vi "Periodic Tasks Cheeto.vi"(8 "error in":errorcluster) -> ()   [LabVIEW 2016]
doc: "This VI runs in parallel to other tasks. It can contain as many user-defined periodic loops as you need. These can carry out PID or other sorts of timed response."
uses:
  Fault_Cluster.ctl
  Faults.ctl
  <vilib>/Platform/TimedLoop/XDataNode/timing_clust.ctl
  <vilib>/Platform/TimedLoop/XDataNode/nitl_modes.ctl
  <vilib>/Platform/TimedLoop/XDataNode/wakeup.ctl
  <vilib>/Rock Robotics/SystemInterfaces/DIO/FPGA_DIOChannel.ctl
  <userlib>/836-libraries/Drive/Drive_Code/Drive_Code_Support/Drive_Code_PID_Bundle.ctl
  <vilib>/Rock Robotics/WPI/ThirdParty/CanMotor/TalonSRX/WPI_CANTalonSRX_APIFeedbackSelect.ctl
  <vilib>/Rock Robotics/WPI/ThirdParty/CanMotor/TalonSRX/WPI_CANTalonSRX_APIControlMode.ctl
  <vilib>/Rock Robotics/WPI/Utilities/WPI_GetSetVariantRefNum.vi
  <vilib>/platform/TimedLoop/XDataNode/XDataNode.xnode
  <vilib>/Platform/TimedLoop/XDataNode/XDNodeRunTimeDep.lvlib
panel:
  out "TurretLate?":bool
  out "Motor Output":dbl=-0.0
  out "Finished Late? [i-1]":bool
  in  "Period":i64=50
  in  "Log Top":bool
  out "Bot Current 2":dbl(graph)=3.75
  in  "Bottom Shooter Wheel Tab":T1(tab)=enum."Turret"
  in  "Tab Control 3":enum32{"TBH", "PID(F)"}(tab)
  in  "Bot Average":u8=10 min=1 max=128
  in  "Bot Min Rate":dbl=20.0
  in  "Bot tbh Gain":dbl
  in  "Enc Counts 3":dbl=4096.0
  in  "FF":bool=TRUE
  out "State":bool=TRUE
  out "Iter":i32=18978
  in  "delay":i32=30
  in  "FF Gain":dbl=0.000182 format="%#_13g"
  in  "Ramp Rate 3":dbl
  in  "I Zone 3":dbl
  in  "F 3":dbl=0.0288
  in  "D 3":dbl=5.0
  in  "I 3":dbl=0.001
  in  "P 3":dbl=0.19
  in  "Rev FB Sensor":bool=TRUE
  in  "Enc Counts":dbl=4096.0
  out "Bot Response":cluster{"Bot Cntrl":dbl, dbl}(graph)={"Bot Cntrl"=0.0, 2145.6268149735524}
  in  "Bot Cntrl":dbl(knob)=2145.6268149735524 scale=0.0..5700.0
  in  "BotInvert":bool=TRUE
  in  "Bot Period":i64=15
  in  "Disable Bottom":bool
  out "Bot Late?":bool
  in  "Bot Tol":dbl=25.0 format="%#_13g"
  out "RPM High .":bool
  out "RPM Low .":bool=TRUE
  out "1 RPM .":bool
  out "5 RPM .":bool
  out "2 RPM .":bool
  out "8 RPM .":bool
  out "7 RPM .":bool
  out "6 RPM .":bool
  out "4 RPM .":bool
  out "3 RPM .":bool
  out "RPM Steady? 2":bool
  in  "Open?":bool=TRUE
  out "Bot Cntrl .":dbl=2145.6268149735524
  in  "Log Bot Current?":bool
  out "Max Bot":dbl=0.29296875
  in  "reset bot":bool
  out "Min Bot":dbl=-0.146484375
  out "Stopped":bool=TRUE
  out "Bot Dist":dbl=67108856.0
  in  "Open Loop Cntrl":dbl(knob)=0.0014346101200435335 scale=-1.0..1.0
  out "Tgrd 2":bool
  out "cnt 2":i16=90
  in  "Arm2":bool=TRUE
  in  "Trig2":dbl=40.0
  in  "Len2":i16=90
  in  "Reset2":bool
  out "State2":i32
  out "File Delete Checking":string
  in  "LogTR":bool
  in  "LogTL":bool
  in  "LogBL":bool
  in  "LogBR":bool
  in  "TR":T2 {"Severity" max=10}
  in  "BR":T2 {"Severity" max=10}
  in  "BL":T2 {"Severity" max=10}
  in  "TL":T2 {"Severity" max=10}
  out "Turret":cluster{"Double":dbl, "desired Angle":dbl}(graph)={"Double"=0.29942691101875774, "desired Angle"=0.0}
  in  "Invert Turret":bool
  in  "Turret Max Speed":dbl(knob)=0.618529087034838 scale=0.0..1.0
  in  "SoftStop":bool=TRUE
  in  "correlation":bool
  out "At Lo":bool
  out "At Hi":bool=TRUE
  in  "Lo Limit":dbl=-70.0
  in  "Hi Limit":dbl=40.0
  in  "Speed near Limit":dbl=0.2
  in  "Near Limit":dbl=40.0
  out "Motor Out":dbl
  out "Angle":dbl
  in  "PID gains":T4={"proportional gain (Kc)"=0.02, "integral time (Ti, min)"=0.0, "derivative time (Td, min)"=0.001} {"derivative time (Td, min)" format="%.3f"; "integral time (Ti, min)" format="%.8f"; "proportional gain (Kc)" format="%.8f"}
  in  "output range":cluster{"output high":dbl, "output low":dbl}={"output high"=1.0, "output low"=-1.0}
  in  "shooter range":dbl=100.0 format="%#_13g"
  in  "Softstop":dbl
  in  "desired Angle":dbl(slide) scale=-100.0..90.0
  in  "Out Bound":dbl=100.0
  in  "Track Target":bool
  in  "Soft Stop Period":dbl(knob) scale=0.0..1.0
  in  "Manual":bool=TRUE
  in  "Soft Stops":T5={"Motor Power"=0.0, "Time to Stop"=0.0, "Hi Limit"=95.0, "Lo Limit"=-90.0, "Speed Near Limit"=0.15, "Near Limit"=35.0}
  in  "Tolerance":dbl
  out "TtR":dbl
  out "Tgrd 3":bool
  out "cnt 3":i16=90
  in  "Arm 2":bool=TRUE
  in  "Trig 2":dbl=20.0
  in  "Len 2":i16=90
  in  "Reset1 2":bool
  out "State1 2":i32
  in  "Invert Primer":bool
  in  "Primer Max Speed":dbl(knob)=1.0 scale=0.0..1.0
  in  "Invert Agitator":bool
  in  "Agitator Max Speed":dbl(knob)=1.0 scale=0.0..1.0
  in  "Invert Intake":bool
  in  "Intake Speed":dbl(knob)=1.0 scale=0.0..1.0
  out "Roll":dbl(graph)=-2.653997926222683
  out "Pitch":dbl(graph)=0.9060832058624935
  out "Yaw":dbl(graph)=64.04836303793759
  out "Yaw Alt":dbl(graph)=1.0254433926321722
  out "Pitch Alt":dbl(graph)=3.179870559290271
  out "Roll Alt":dbl(graph)=14.748416919967577
  in  "Top Shooter Wheel Tab":T6(tab)=enum."Control"
  in  "Tab Control 2":enum32{"TBH", "PID(F)"}(tab)=enum."PID(F)"
  in  "switch pnt":dbl=2800.0
  in  "Top Gain (lower)":dbl=6e-06
  in  "Top Gain (upper)":dbl=2e-05
  in  "Top Min Rate":dbl=20.0
  in  "Top Average":u8=30 min=1 max=128
  in  "P 2":dbl=0.075 format="%#_8g"
  in  "I 2":dbl=0.001
  in  "D 2":dbl=5.0
  in  "F 2":dbl=0.0132
  in  "I Zone 2":dbl
  in  "Ramp Rate 2":dbl
  in  "Enc Counts 2":dbl=4096.0
  in  "Rev FB Sensor 2":bool=TRUE
  out "Top Cntrl .":dbl=-3139.2166644166086
  in  "Top Cntrl":dbl(knob)=-3139.2166644166086 scale=-7000.0..7000.0
  out "Top Response":cluster{"Top Cntrl":dbl, dbl}(graph)={"Top Cntrl"=0.0, -3139.2166644166086}
  in  "TopInvert":bool
  in  "Top Period":i64=17
  in  "Disable Top":bool
  out "RPM Steady? Top":bool
  out "3 RPM":bool
  out "4 RPM":bool
  out "6 RPM":bool
  out "7 RPM":bool
  out "8 RPM":bool
  out "2 RPM":bool
  out "5 RPM":bool
  out "1 RPM":bool
  out "RPM Low":bool
  out "RPM High":bool=TRUE
  in  "Top Tol":dbl=25.0 format="%#_13g"
  out "Top Late?":bool
  in  "reset top":bool
  out "Max top":dbl=0.43945312499999994
  out "Min Top":dbl=-0.732421875
  out "Stopped 2":bool=TRUE
  out "Top Dist":dbl=-67108864.0
  out "Tgrd":bool
  out "cnt":i16=90
  in  "Arm":bool=TRUE
  in  "Trig":dbl=20.0
  in  "Len":i16=90
  in  "Reset1":bool
  out "State1":i32
  in  "Top Open":bool=TRUE
  in  "Output":dbl(knob) scale=0.0..10.0
  out "appended path":path
  out "TDMS Name":string="Shooter Log"
  in  "Log to USB?":bool
  in  "TDMS Name 2":string="Shooter Log"
  out "File Creation Loop Iteration":i32
  in  "Burst 2":i32=75
  out "Save Drive 2":bool=TRUE
  out "Save Drive":bool
  in  "Burst":i32=75
  in  "loop period (ms) 2":u32=200
  out "Bot Current":dbl(graph)=3.0
  out "Top Current":dbl(graph)
  in  "Bot Channel":i32=14
  in  "Top Channel":i32=13
  in  "Bot Channel 2":i32=2
  # "Start"
  # "Top Wheel"
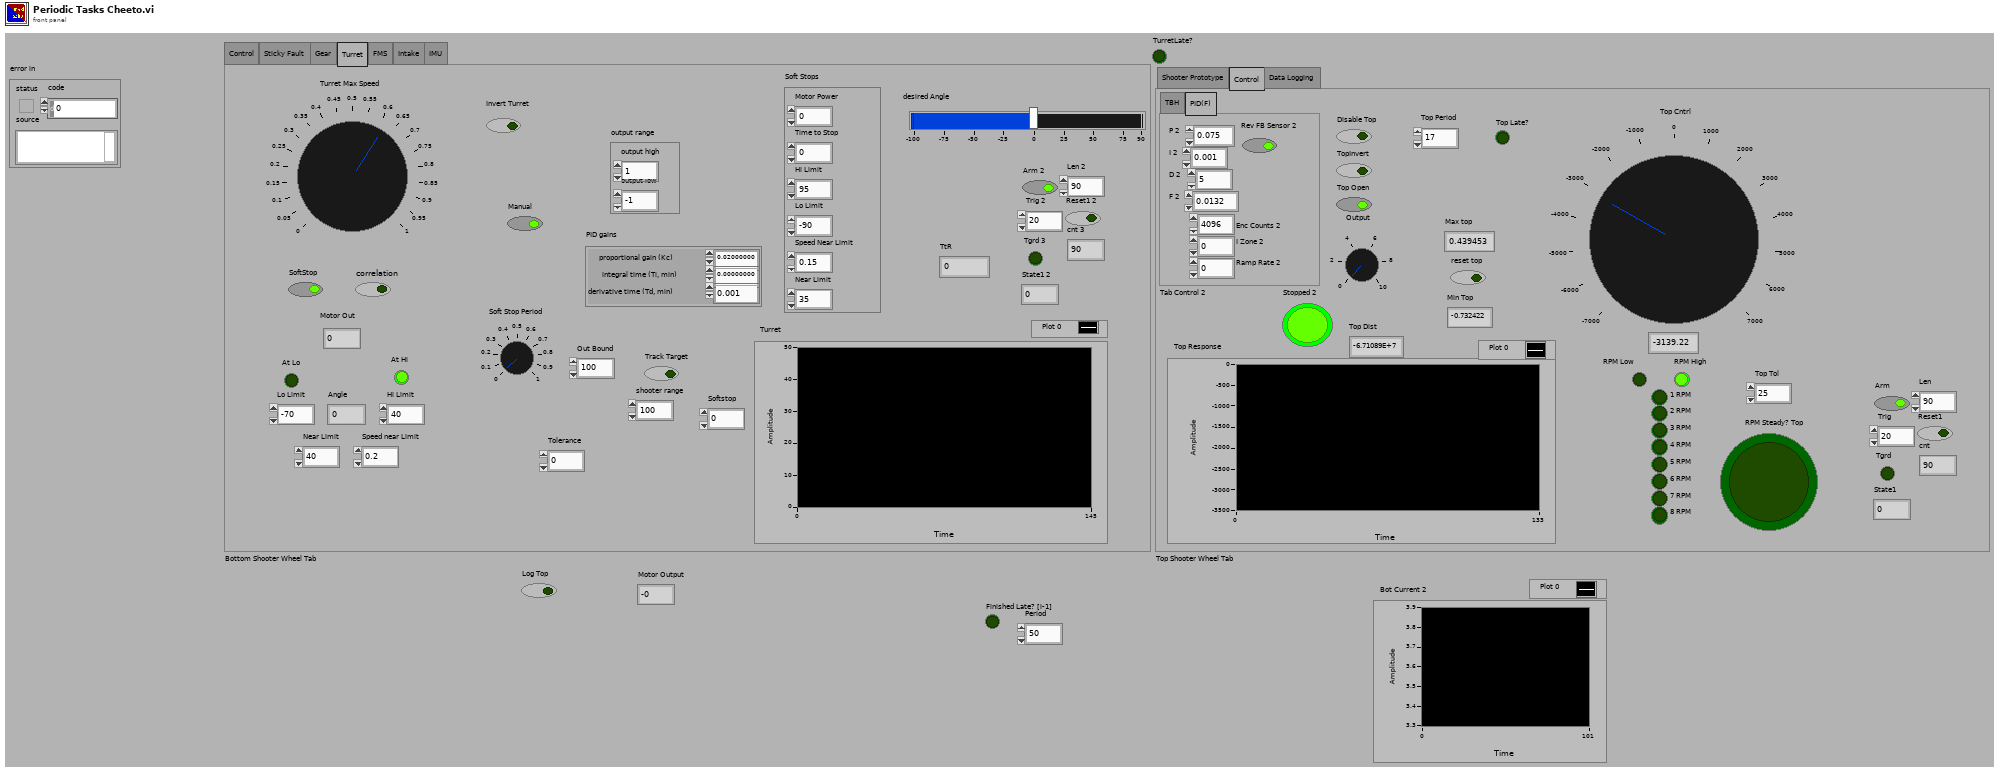
[diagram p1: front panel]
types:
  T1 = enum32{"Control", "Sticky Fault", "Gear", "Turret", "FMS", "Intake", "IMU"}
  T2 = typedef "Fault_Cluster.ctl" = cluster{"Error Code":T3, "Severity":u32, "Message":string, "Origin":string}
  T3 = typedef "Faults.ctl" = enum16{"Boiler Target Lost", "Gerar Target Lost", "Body IMU Fault", "Turret IMU Fault"}
  T4 = cluster{"proportional gain (Kc)":dbl, "integral time (Ti, min)":dbl, "derivative time (Td, min)":dbl}
  T5 = cluster{"Motor Power":dbl, "Time to Stop":dbl, "Hi Limit":dbl, "Lo Limit":dbl, "Speed Near Limit":dbl, "Near Limit":dbl}
  T6 = enum32{"Shooter Prototype", "Control", "Data Logging"}
  T7 = typedef "FPGA_DIOChannel.ctl" = enum8{"DIO 0", "DIO 1", "DIO 2", "DIO 3", "DIO 4", "DIO 5", "DIO 6", "DIO 7", "DIO 8", "DIO 9", "DIO MXP 0", "DIO MXP 1", "DIO MXP 2", "DIO MXP 3", "DIO MXP 4", "DIO MXP 5", "DIO MXP 6", "DIO MXP 7", "DIO MXP 8", "DIO MXP 9", "DIO MXP 10", "DIO MXP 11", "DIO MXP 12", "DIO MXP 13", "DIO MXP 14", "DIO MXP 15", "SPI Port CS1", "SPI Port CS2", "SPI Port CS3", "SPI Port MISO", "SPI Port MOSI", "Invalid"}
  T8 = typedef "XDNodeRunTimeDep.lvlib/timing_clust.ctl" = cluster{"Expected End [f-1]":u64, "Actual End [f-1]":u64, "Finished Late? [f-1]":bool, "Expected End [i-1]":u64, "Actual End [i-1]":u64, "Finished Late? [i-1]":bool, "Expected Start [i]":u64, "Actual Start [i]":u64, "Expected Start [f]":u64, "Actual Start [f]":u64, "Source Name":string, "Structure Name":string, "Period":i64, "Deadline":i64, "Offset":i64, "Start":i64, "Priority":i32, "Timeout":i32, "Mode":T9, "Wakeup Reason":T10, "Error":errorcluster, "Source Type":string, "Secondary Source Type":string, "Global End Time":u64, "Global Start Time":u64, "Frame Duration":u64, "Iteration Duration":u64, "Assigned CPU":i32, "I/O Scan Engine Mode":u32}
  T9 = typedef "XDNodeRunTimeDep.lvlib/nitl_modes.ctl" = enum32{"No Change", "Process missed periods, maintain original phase", "Discard missed periods, maintain original phase", "Process missed periods, ignore original phase", "Discard missed periods, ignore original phase"}
  T10 = typedef "XDNodeRunTimeDep.lvlib/wakeup.ctl" = enum32{"Normal", "Aborted", "Asynchronous wakeup", "Timing source error", "Timed loop error", "Timeout"}
  T11 = typedef "Fault_Fifos.ctl" = cluster{"Error Code":refnum<k33>, "Severity":refnum<k33>, "Burst":refnum<k4>, "BurstSize":u32, "Timing Notifier":refnum<notifier>, "Timing Trigger":u16}
  T12 = enum16{"open", "open or create", "create or replace", "create", "open (read-only)"}
  T13 = typedef "WPI_MotorControlDeviceRef.ctl" = cluster{"DeviceStatus":errorcluster, "Type":T14, "PWM":cluster{"PWM Channel":T15, "DeadBand":T16}, "CAN":cluster{"Device Number":u8, "SetOutput VI Ref":variant, "GetOutput VI Ref":variant, "Enable VI Ref":variant, "Disable VI Ref":variant, "Data":variant}, "Invert":bool}
  T14 = typedef "WPI_MotorControlType.ctl" = enum16{"PWM", "CAN"}
  T15 = typedef "FPGA_DIOPWMChannel.ctl" = enum8{"PWM 0", "PWM 1", "PWM 2", "PWM 3", "PWM 4", "PWM 5", "PWM 6", "PWM 7", "PWM 8", "PWM 9", "PWM MXP 0", "PWM MXP 1", "PWM MXP 2", "PWM MXP 3", "PWM MXP 4", "PWM MXP 5", "PWM MXP 6", "PWM MXP 7", "PWM MXP 8", "PWM MXP 9", "Invalid"}
  T16 = typedef "WPI_PWMDeadband.ctl" = cluster{"Name":string, "maxPositivePwm":i32, "minPositivePwm":i32, "centerPwm":i32, "maxNegativePwm":i32, "minNegativePwm":i32, "angularRange":u16}
  T17 = typedef "WPI_EncoderDevRef.ctl" = cluster{"DevStatus":errorcluster, "EncoderIndex":T18, "CounterIndex":T19, "DistancePerCount":dbl, "Decoding Type":T20}
  T18 = typedef "FPGA_EncoderIdx.ctl" = enum8{"Enc 0", "Enc 1", "Enc 2", "Enc 3", "Enc 4", "Enc 5", "Enc 6", "Enc 7", "Invalid"}
  T19 = typedef "FPGA_CounterCtrSystemIndex.ctl" = enum8{"Ctr 0", "Ctr 1", "Ctr 2", "Ctr 3", "Ctr 4", "Ctr 5", "Ctr 6", "Ctr 7", "Invalid"}
  T20 = typedef "WPI_EncoderType.ctl" = enum16{"1x", "2x", "4x"}
  T21 = typedef "WPI_CANTalonSRX_APIFeedbackSelect.ctl" = enum16{"Digital Quadrature Encoder", "Analog Potentiometer", "Analog Encoder", "Count on Quad-A (Rising-Edge)", "Count on Quad-A (Falling-Edge)", "CTR Magnetic Enc (Absolute)", "CTR Magnetic Enc (Relative)", "Pulse Width"}
  T22 = typedef "WPI_CANTalonSRX_APIControlMode.ctl" = enum8{"Percent VBus", "Speed", "Position", "Slave", "Unchanged / Invalid", "Voltage Compensation", "Current", "Motion Profile", "Motion Magic"}
  T23 = typedef "WPI_CANTalonSRX_GlobalStatus.ctl" = cluster{"Applied Throttle":dbl, "Module Enabled":bool, "CAN Error":errorcluster, "Closed Loop Error":dbl, "Forward Limit Switch Closed":bool, "Reverse Limit Switch Closed":bool, "Sensor Position":dbl, "Sensor Velocity":dbl, "Current":dbl, "Sticky Fault - Over Temp":bool, "Sticky Fault - Under Voltage":bool, "Sticky Fault - Forward Limit":bool, "Sticky Fault - Reverse Limit":bool, "Sticky Fault - Forward Soft Limit":bool, "Sticky Fault - Reverse Soft Limit":bool, "Brake is Enabled":bool, "Encoder Position":dbl, "Encoder Velocity":dbl, "Encoder Index Count":dbl, "Encoder A Pin State":bool, "Encoder B Pin State":bool, "Encoder Index Pin State":bool, "Analog In":dbl, "Analog In Velocity":dbl, "Temperature (C)":dbl, "Battery Voltage":dbl, "Control 5 Is Supported":bool, "Current Profile Slot Select":dbl, "Pos Div 8":bool, "Vel Div 4":bool, "Pulse Width Position":i32, "Pulse Width Velocity":i32, "Pulse Width Rise To Rise (us)":i32, "Pulse Width Rise To Fall (us)":i32, "Mot Prof Active Is Under Run":bool, "Mot Prof Active Has Under Run":bool, "Mot Prof Active Is Last":bool, "Mot Prof Active Velocity Only":bool, "Mot Prof Active Is Valid":bool, "Mot Prof Buffer Is Full":bool, "Mot Prof Active Profile Slot Select":i32, "Mot Prof NextID":i32, "Mot Prof Count":i32, "Mot Prof Active Velocity":dbl, "Mot Prof Active Position":dbl, "Mot Prof Output Enable":i32}
  T24 = typedef "WPI_JoystickDevRef.ctl" = cluster{"Device":T25}
  T25 = typedef "WPI_JoystickDeviceEnum.ctl" = enum16{"USB 0", "USB 1", "USB 2", "USB 3", "USB 4", "USB 5"}
  T26 = typedef "WPI_DigitalInputDevRef.ctl" = cluster{"DevStatus":errorcluster, "DIO Channel":T7}
  T27 = typedef "WPI_I2CDevRef.ctl" = cluster{"DevStatus":errorcluster, "Device Address":u8, "Handle":i32, "I2C Bus":T28}
  T28 = typedef "i2c_bus.ctl" = enum16{"I2C On-Board", "I2C MXP", "Invalid"}
  T29 = cluster{"Yaw":dbl, "Roll":dbl, "Pitch":dbl, "Yaw Wind":dbl, "Roll Wind":dbl, "Pitch Wind":dbl}
  T30 = typedef "WPI_RobotDriveDevRef.ctl" = cluster{"DevStatus":errorcluster, "Motors[]":T13[], "Square Inputs":bool, "Max Output":dbl}
  T31 = typedef "Drive_Code_Bundle.ctl" = cluster{"Sensor Data":T32, "Drive Command rt fifo":refnum<k33>, "Logging Data":refnum<k33>, "PID Update":refnum<notifier>}
  T32 = typedef "Sensor_Cluster.ctl" = cluster{"Gyro Data":cluster{"Gyro RT FIFO":refnum<k33>, "Gyro Current":dbl, "Gyro Hold":dbl}, "Encoder Data":cluster{"Encoder RT FIFO":refnum<k33>, "Encoder Current":dbl, "Encoder Hold":dbl}, "Camera Data":cluster{"Camera RT FIFO":refnum<k33>, "Camera Current":T33}}
  T33 = typedef "Camera_Cluster.ctl" = cluster{" Angle":dbl, "Valid":bool}
  T34 = typedef "Drive_Code_PID_Bundle.ctl" = cluster{"Yaw, Driving Straight":cluster{"proportional gain (Kc)":dbl, "integral time (Ti, min)":dbl, "derivative time (Td, min)":dbl}, "Yaw, Holding Still":cluster{"proportional gain (Kc)":dbl, "integral time (Ti, min)":dbl, "derivative time (Td, min)":dbl}, "Distance, Driving Straight":cluster{"proportional gain (Kc)":dbl, "integral time (Ti, min)":dbl, "derivative time (Td, min)":dbl}, "Distance, Holding Still":cluster{"proportional gain (Kc)":dbl, "integral time (Ti, min)":dbl, "derivative time (Td, min)":dbl}}
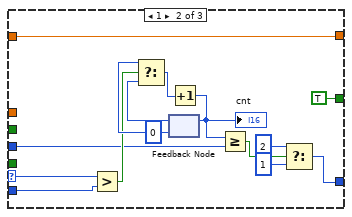
[diagram p3: hidden frame]
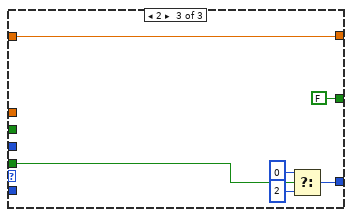
[diagram p4: hidden frame]
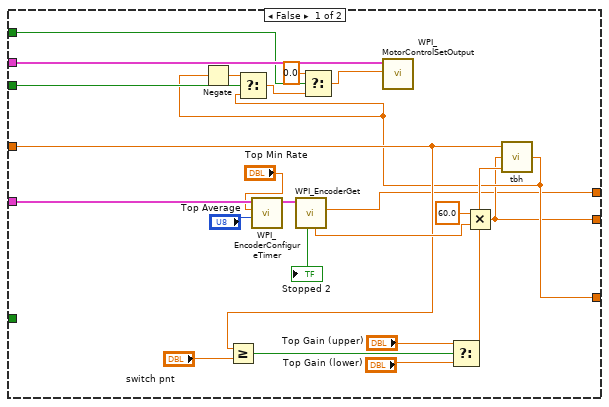
[diagram p6: hidden frame]
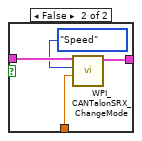
[diagram p7: hidden frame]
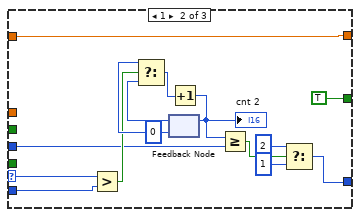
[diagram p9: hidden frame]
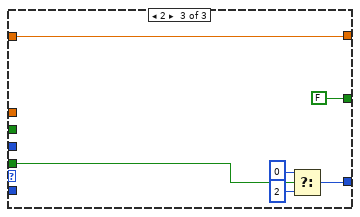
[diagram p10: hidden frame]
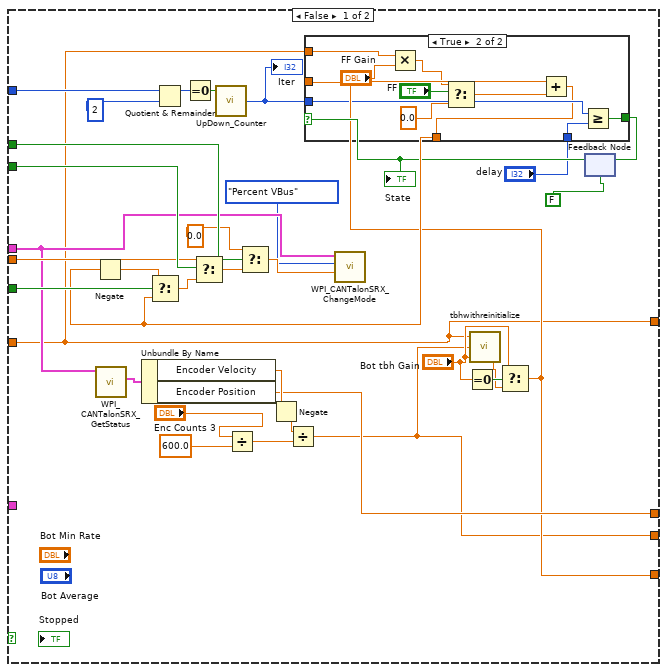
[diagram p11: hidden frame]
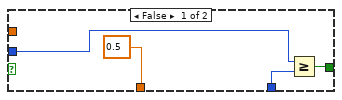
[diagram p12: hidden frame]
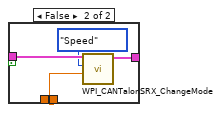
[diagram p14: hidden frame]
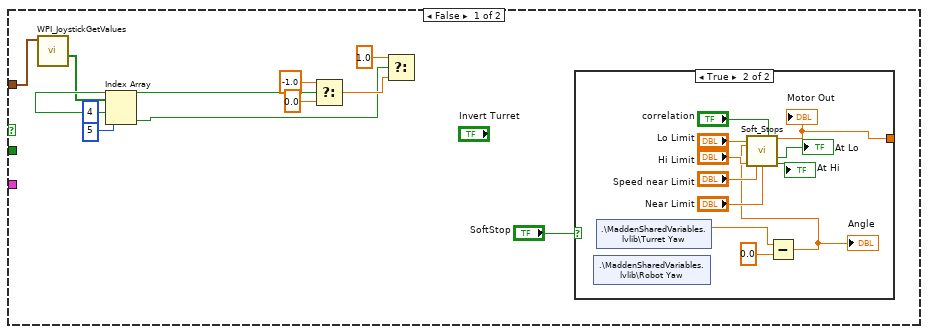
[diagram p16: hidden frame]
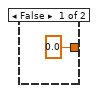
[diagram p17: hidden frame]
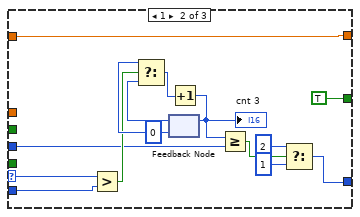
[diagram p19: hidden frame]
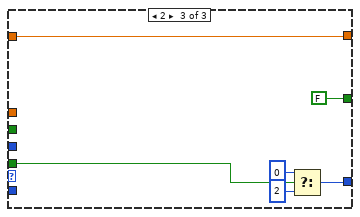
[diagram p20: hidden frame]
diagram:
  # "Drive FIFO Setup"
  # "rising edges\none channel only\nspeed control"
  n1 = disable-structure shown="Disabled" {
    disable-tunnel: [w55 _] -> w48
    frame Disabled {
      n2 = while {
        tunnel: [w68] -> w55
        tunnel: "Log to USB?" -> [w57]
        tunnel: "TDMS Name 2" -> [w56]
        i -> [w72]
        stop <- w69 continue-if-true
        # "Can tweak this such that it doesn't start until Time > 1970"
        n3 = Current VI's Path() -> (path=w67:path)
        n4 = Strip Path(path=w67) -> (stripped path=w61:path)  [unwired: 1 out]
        n5 = String To Path(string="~/") -> (path=w65:path)
        n6 = Select(t=w65, s=w57, f=w61) -> (s? t:f=w66:path)
        n7 = Get Date/Time In Seconds() -> (seconds since 1Jan1904=w74:timestamp)
        n8 = case shown="False" w57 {
          selector: w57 -> [w80 _]
          tunnel: w66 -> [w79 w85]
          tunnel: [w79 w82] -> w63
          tunnel: [w80 w81] -> w60
          frame False {
          }
          frame True {
            n9 = Build Path(base path=w85, name or relative path="LogFiles") -> (appended path=w84:path)
            n10 = call <vilib>:"Check if File or Folder Exists.vi"("path"=w84) -> ("file or folder exists?"=w88:bool, "dup path"=w87:path)  [unwired: 8 in, 1 out]
            n11 = case shown="False" w88 {
              tunnel: [w90 w91] -> w83
              tunnel: w87 -> [w89 w91]
              frame False {
                n12 = Create Folder(path (use dialog)=w89) -> (created path=w90:path)  [unwired: 2 in, 2 out]
              }
              frame True {
              }
            }
            n13 = call <vilib>:"Check if File or Folder Exists.vi"("path"=w83) -> ("file or folder exists?"=w81:bool, "dup path"=w82:path)  [unwired: 8 in, 1 out]
          }
        }
        n14 = Format Date/Time String(time format string (%c)="%m-%#d-%Y %H%M", seconds (now)=w74, UTC format=FALSE) -> (date/time string=w77:string)
        n15 = Number To Hexadecimal String(1:i16 4 ("width (-)"), 2:w72) -> (0:w70:string)
        n16 = Concatenate Strings(w56, w77, w70, ".tdms" ("string")) -> (w78:string)
        n17 = case shown="True" w60 {
          tunnel: w61 -> [w96 w101]
          tunnel: [w92 w101] -> w59
          frame False {
            n18 = Build Path(base path=w96, name or relative path="LogFiles") -> (appended path=w93:path)
            n19 = call <vilib>:"Check if File or Folder Exists.vi"("path"=w93) -> ("file or folder exists?"=w94:bool, "dup path"=w95:path)  [unwired: 8 in, 1 out]
            n20 = case shown="False" w94 {
              tunnel: [w99 w100] -> w92
              tunnel: w95 -> [w98 w100]
              frame False {
                n21 = Create Folder(path (use dialog)=w98) -> (created path=w99:path)  [unwired: 2 in, 2 out]
              }
              frame True {
              }
            }
          }
          frame True {
          }
        }
        n22 = Select(t=w63, s=w60, f=w59) -> (s? t:f=w62:path)
        n23 = Build Path(base path=w62, name or relative path=w78) -> (appended path=w68:path)
        n24 = call <vilib>:"Check if File or Folder Exists.vi"("path"=w68) -> ("file or folder exists?"=w69:bool)  [unwired: 8 in, 2 out]
        n25 = Wait (ms)(milliseconds to wait=u32 1 ("millisecond multiple")) -> ()  [unwired: 1 out]
        "File Creation Loop Iteration" <- w72
      }
      n26 = disable-structure shown="Disabled" {
        frame Disabled {
          w109 = i64 50 ("Period")
          # "needs testing"
          # "Periodic Data Log Setup"
          n27 = Obtain Notifier(name (unnamed)="Timing", notification data type=u16 0) -> (notifier out=w105:refnum<notifier>)  [unwired: 2 in, 2 out]
          n28 = call "OpenFaultLogger.vi"("Timing Trigger"=u16 1, "Timing Notifier"=w105, "BurstSize"=u32 4, "BufferSize"=u32 100) -> ("FaultDevRef"=w102:T11)  [unwired: 7 in]
          n29 = node-c288(w109) -> (w118:T8)  [unwired: 3 in]
          n30 = node-c288(w109) -> (w112:T8)  [unwired: 3 in]
          n31 = timed-loop {
            timing: w118 -> [_]
            timing-out: [_] -> w117
            tunnel: w102 -> [w151]
            stop <- FALSE stop-if-true
            n32 = node-c288() -> ()  [unwired: 1 in, 1 out]
            n33 = call "WriteFault.vi"("Fault"="TL", "FaultDevRef"=w151) -> ()  [unwired: 1 in]
            n34 = while {
              stop <- "LogTL" stop-if-true
            }
            n35 = node-c288() -> ()  [unwired: 1 in, 1 out]
          }
          n36 = timed-loop {
            timing: w112 -> [_]
            timing-out: [_] -> w111
            tunnel: w102 -> [w121]
            stop <- FALSE stop-if-true
            n37 = node-c288() -> ()  [unwired: 1 in, 1 out]
            n38 = while {
              stop <- "LogBL" stop-if-true
            }
            n39 = call "WriteFault.vi"("Fault"="BL", "FaultDevRef"=w121) -> ()  [unwired: 1 in]
            n40 = node-c288() -> ()  [unwired: 1 in, 1 out]
          }
          n41 = node-c288(w117) -> ()  [unwired: 1 out]
          n42 = node-c288(w111) -> ()  [unwired: 1 out]
          n43 = call "FaultLogger.vi"("Period"=i64 20, "FaultDevRef"=w102) -> ()  [unwired: 10 in]
          n44 = node-c288(w109) -> (w114:T8)  [unwired: 3 in]
          n45 = node-c288(w109) -> (w116:T8)  [unwired: 3 in]
          n46 = timed-loop {
            timing: w114 -> [_]
            timing-out: [_] -> w113
            tunnel: w102 -> [w131]
            stop <- FALSE stop-if-true
            n47 = node-c288() -> ()  [unwired: 1 in, 1 out]
            n48 = while {
              stop <- "LogBR" stop-if-true
            }
            n49 = call "WriteFault.vi"("Fault"="BR", "FaultDevRef"=w131) -> ()  [unwired: 1 in]
            n50 = node-c288() -> ()  [unwired: 1 in, 1 out]
          }
          n51 = timed-loop {
            timing: w116 -> [_]
            timing-out: [_] -> w115
            tunnel: w102 -> [w141]
            stop <- FALSE stop-if-true
            n52 = node-c288() -> ()  [unwired: 1 in, 1 out]
            n53 = call "WriteFault.vi"("Fault"="TR", "FaultDevRef"=w141) -> ()  [unwired: 1 in]
            n54 = while {
              stop <- "LogTR" stop-if-true
            }
            n55 = node-c288() -> ()  [unwired: 1 in, 1 out]
          }
          n56 = node-c288(w113) -> ()  [unwired: 1 out]
          n57 = node-c288(w115) -> ()  [unwired: 1 out]
        }
        frame Enabled {
        }
      }
    }
    frame Enabled {
    }
  }
  "appended path" <- w48
  n58 = disable-structure shown="Disabled" {
    frame Disabled {
      n59 = node-c288(i64 100 ("Period")) -> (w161:T8)  [unwired: 3 in]
      n60 = timed-loop {
        timing: w161 -> [_]
        timing-out: [_] -> w160
        stop <- FALSE stop-if-true
        w162 = 1.0 ("Secondary True Time")
        # "needs verified"
        # "0: delete file\n1: ask if sure\n2: don't do anything"
        # "Sticky Fault File Deletion"
        n61 = node-c288() -> ()  [unwired: 1 in, 1 out]
        n62 = call <vilib>:"WPI_UtilitiesFRC ReadUserButton.vi"() -> ("User Button"=w176:bool)  [unwired: 10 in, 1 out]
        n63 = call <userlib>:"BoolConfirmCheck.vi"("False Time"=3.0, "Secondary True Time"=w162, "Inital True Time"=5.0, "Signal"=w176) -> ("First Time Met"=w172:bool, "Out Signal"=w173:bool)
        n64 = call <userlib>:"Pulse_Stretch_&_Delay.vi"("In"=w172, "Width (sec)"=w162) -> ("Out"=w164:bool)  [unwired: 3 in]
        n65 = call <userlib>:"Pulse_Stretch_&_Delay.vi"("In"=w173, "Width (sec)"=w162) -> ("Out"=w163:bool)  [unwired: 3 in]
        n66 = Select(t=1, s=w164, f=2) -> (s? t:f=w168:i32)
        n67 = Select(t=0, s=w163, f=w168) -> (s? t:f=w166:i32)
        n68 = case shown="1" w166 {
          tunnel: ["File Deleted" "Ask if Sure" "Nothing Done To File"] -> w165
          frame 0 {
          }
          frame 1 {
          }
          frame 2, Default {
          }
        }
        "File Delete Checking" <- w165
        n69 = node-c288() -> ()  [unwired: 1 in, 1 out]
      }
      n70 = node-c288(w160) -> ()  [unwired: 1 out]
    }
    frame Enabled {
    }
  }
  n71 = disable-structure shown="Disabled" {
    disable-tunnel: w48 -> [w187 _]
    frame Disabled {
      w198 = 9 ("dimension size")
      # "Size of Drive Log"
      # "13"
      n72 = TDMS Open(6:TRUE ("disable buffering? (T)"), 7:enum16{"1.0", "2.0"}."2.0" ("file format version (2.0)"), 10:T12."open or create" ("operation (0:open)"), 11:w187) -> (3:w192:refnum<k34>)  [unwired: 3 in, 1 out]
      n73 = Initialize Array(0.0, w198) -> (w188:dbl[])
      n74 = To Unsigned Long Integer(number=w198) -> (unsigned 32bit integer=w199:u32)
      n75 = RT FIFO Create(0:"Drive FIFO" ("name (unnamed)"), 1:w188, 4:u32 100 ("size (10)"), 6:w199) -> (8:w190:refnum<k33>)  [unwired: 4 in, 2 out]
      n76 = while "Drive Logging Loop" {
        tunnel: w190 -> [w239]
        tunnel: w188 -> [w238]
        tunnel: w192 -> [w237]
        stop <- FALSE stop-if-true
        n77 = local read "Save Drive 2"() -> (w235:bool)
        n78 = local read "Burst 2"() -> (w233:i32)
        n79 = disable-structure shown="Disabled" {
          disable-tunnel: w239 -> [w244 _]
          disable-tunnel: w238 -> [w243 _]
          disable-tunnel: w237 -> [w242 _]
          disable-tunnel: w235 -> [w241 _]
          disable-tunnel: w233 -> [w240 _]
          frame Disabled {
            n80 = call "Drive Data Logger.vi"("Save"=w241, "Array"=w243, "Burst"=w240, "rt fifo"=w244, "TDMS Refnum"=w242) -> ()  [unwired: 7 in]
          }
          frame Enabled {
          }
        }
        n81 = Wait (ms)(milliseconds to wait="loop period (ms) 2") -> ()  [unwired: 1 out]
      }
      n82 = Get Date/Time In Seconds() -> (seconds since 1Jan1904=w191:timestamp)
      n83 = To Double Precision Float(number=w191) -> (double precision float=w189:dbl)
      n84 = while {
        tunnel: w190 -> [w212]
        tunnel: w188 -> [w211]
        tunnel: w189 -> [w210]
        stop <- FALSE stop-if-true
        n85 = shared-variable ".\\Untitled Library 1.lvlib\\Control Signal1"() -> (w209:dbl)  [unwired: 1 in, 1 out]
        n86 = shared-variable ".\\Untitled Library 1.lvlib\\Current1"() -> (w208:dbl)  [unwired: 1 in, 1 out]
        n87 = shared-variable ".\\Untitled Library 1.lvlib\\Rpm1"() -> (w207:dbl)  [unwired: 1 in, 1 out]
        n88 = shared-variable ".\\Untitled Library 1.lvlib\\Control Signal2"() -> (w206:dbl)  [unwired: 1 in, 1 out]
        n89 = shared-variable ".\\Untitled Library 1.lvlib\\Current2"() -> (w205:dbl)  [unwired: 1 in, 1 out]
        n90 = shared-variable ".\\Untitled Library 1.lvlib\\Rpm2"() -> (w204:dbl)  [unwired: 1 in, 1 out]
        n91 = shared-variable ".\\Untitled Library 1.lvlib\\Current3"() -> (w200:dbl)  [unwired: 1 in, 1 out]
        n92 = case shown="True" TRUE {
          tunnel: w211 -> [_ w228]
          tunnel: w210 -> [_ w227]
          tunnel: w212 -> [_ w226]
          tunnel: w209 -> [_ w221]
          tunnel: w208 -> [_ w220]
          tunnel: w207 -> [_ w219]
          tunnel: w206 -> [_ w218]
          tunnel: w205 -> [_ w217]
          tunnel: w204 -> [_ w216]
          tunnel: w200 -> [_ w214]
          frame False {
          }
          frame True {
            n93 = Get Date/Time In Seconds() -> (seconds since 1Jan1904=w231:timestamp)
            n94 = To Double Precision Float(number=w231) -> (double precision float=w232:dbl)
            n95 = Subtract(x=w232, y=w227) -> (x-y=w222:dbl)
            n96 = feedback #1(u32 0 ("# elements")) -> (w215:u32)
            n97 = Replace Array Subset(array=w228, new element #1=w222, new element #2=w221, new element #3=w220, new element #4=w219, new element #5=w218, new element #6=w217, new element #7=w216, new element #8=w214, new element #9=w215) -> (w229:dbl[])  [unwired: 9 in]
            n98 = RT FIFO Write(0:w226, 1:w229) -> (7:w225:u32)  [unwired: 3 in, 3 out]
            n99 = feedback-in #1(w225) -> ()
            n100 = Greater?(x=w225, y="Burst 2") -> (0:→"Save Drive 2":bool)
          }
        }
        n101 = Wait (ms)(milliseconds to wait=u32 20) -> ()  [unwired: 1 out]
        n102 = Wait (ms)(milliseconds to wait=u32 40) -> ()  [unwired: 1 out]
      }
    }
    frame Enabled {
    }
  }
  n103 = call <vilib>:"WPI_MotorControlRefNum Registry Get.vi"("refnum name"="TopMotor") -> ("MotorControlDevRef"=w1:T13)  [unwired: 9 in, 1 out]
  n104 = call <vilib>:"WPI_EncoderRefNum Registry Get.vi"("refnum name"="TopWheelSpeed") -> ("EncoderDevRef"=w2:T17)  [unwired: 9 in, 1 out]
  n105 = node-c288() -> (w6:T8)  [unwired: 5 in]
  n106 = timed-loop {
    timing: w6 -> [_]
    timing-out: [_] -> w5
    tunnel: w2 -> [w300]
    tunnel: w1 -> [w302]
    stop <- FALSE stop-if-true
    w261 = 0.0
    n107 = node-c288() -> (→"Top Late?":bool)  [unwired: 1 in, 1 out]
    n108 = case shown="True" "Log Top" {
      frame False {
      }
      frame True {
        n109 = call <vilib>:"WPI_Power Get PDP Currents.vi"("PDP Channel"="Top Channel") -> ("current (A)"=w354:dbl)  [unwired: 12 in, 2 out]
        "Top Current" <- w354
        n110 = shared-variable ".\\Untitled Library 1.lvlib\\Current2"(w354) -> ()  [unwired: 1 in, 1 out]
      }
    }
    n111 = case shown="True" TRUE {
      tunnel: w302 -> [w378 w389]
      tunnel: w300 -> [w376 _]
      tunnel: "TopInvert" -> [w373 _]
      tunnel: "Disable Top" -> [w367 _]
      tunnel: "Top Cntrl" -> [w360 w385]
      tunnel: [w359 w387] -> w271
      tunnel: [w357 w379] -> w246
      tunnel: [w356 w388] -> w259
      tunnel: "Top Open" -> [_ w380]
      frame False {
        n112 = Greater Or Equal?(x=w360, y="switch pnt") -> (x >= y?=w361:bool)
        n113 = call <vilib>:"WPI_EncoderConfigureTimer.vi"("Number Samples to Average"="Top Average", "Minimum Rate"="Top Min Rate", "EncoderDevRef"=w376) -> ("EncoderDevRef"=w377:T17)  [unwired: 7 in, 1 out]
        n114 = call <vilib>:"WPI_EncoderGet.vi"("EncoderDevRef"=w377) -> ("Distance"=w356:dbl, "Rate"=w371:dbl, "Stopped"=→"Stopped 2":bool)  [unwired: 5 in, 3 out]
        n115 = Select(t="Top Gain (upper)", s=w361, f="Top Gain (lower)") -> (s? t:f=w363:dbl)
        n116 = Multiply(x=60.0 ("y"), y=w371) -> (x*y=w357:dbl)
        n117 = call "tbh.vi"("Gain"=w363, "Act"=w357, "Cmd"=w360) -> ("Out"=w359:dbl)
        n118 = Negate(x=w359) -> (-x=w372:dbl)
        n119 = Select(t=w372, s=w373, f=w359) -> (s? t:f=w369:dbl)
        n120 = Select(t=0.0, s=w367, f=w369) -> (s? t:f=w368:dbl)
        n121 = call <vilib>:"WPI_MotorControlSetOutput.vi"("Output"=w368, "MotorControlDevRef"=w378) -> ()  [unwired: 7 in, 3 out]
      }
      frame True {
        n122 = call <vilib>:"WPI_CANTalonSRX_SetReference.vi"("Reverse Feedback Sensor"="Rev FB Sensor 2", "Feedback Reference"=WPI_CANTalonSRX_APIFeedbackSelect."Digital Quadrature Encoder", "CAN Talon SRX Ref"=w389) -> ("CAN Talon SRX Ref"=w401:T13)  [unwired: 7 in, 1 out]
        n123 = Divide(x="Enc Counts 2", y=600.0) -> (x/y=w390:dbl)
        n124 = Multiply(x=w390, y=w385) -> (x*y=w383:dbl)
        n125 = call <vilib>:"WPI_CANTalonSRX_SetPID.vi"("CAN Talon SRX Ref"=w401, "Parameter Slot"=u8 0, "P"="P 2", "I"="I 2", "D"="D 2", "F"="F 2", "I Zone"="I Zone 2", "Ramp Rate"="Ramp Rate 2") -> ("CAN Talon SRX Ref"=w403:T13)  [unwired: 6 in, 1 out]
        n126 = Negate(x=w383) -> (-x=w381:dbl)
        n127 = case shown="True" w380 {
          tunnel: w403 -> [w407 w411]
          tunnel: [w406 w410] -> w402
          tunnel: w381 -> [_ w408]
          frame True {
            n128 = call <vilib>:"WPI_CANTalonSRX_ChangeMode.vi"("Output"="Output", "Control Mode"=WPI_CANTalonSRX_APIControlMode."Percent VBus", "CAN Talon SRX Ref"=w407) -> ("CAN Talon SRX Ref"=w406:T13)  [unwired: 7 in, 1 out]
          }
          frame False {
            n129 = call <vilib>:"WPI_CANTalonSRX_ChangeMode.vi"("Output"=w408, "Control Mode"=WPI_CANTalonSRX_APIControlMode."Speed", "CAN Talon SRX Ref"=w411) -> ("CAN Talon SRX Ref"=w410:T13)  [unwired: 7 in, 1 out]
          }
        }
        n130 = call <vilib>:"WPI_CANTalonSRX_GetStatus.vi"("CAN Talon SRX Ref"=w402) -> ("Talon SRX Status"=w400:T23)  [unwired: 8 in, 2 out]
        n131 = Unbundle By Name(w400) -> ("Encoder Velocity"=w386:dbl, "Applied Throttle"=w387:dbl, "Encoder Position"=w388:dbl)
        n132 = Divide(x=w386, y=w390) -> (x/y=w379:dbl)
      }
    }
    "Top Dist" <- w259
    n133 = feedback #2(w261) -> (w269:dbl)
    n134 = Select(t=-inf, s="reset top", f=w269) -> (s? t:f=w268:dbl)
    n135 = Max & Min(x=w246, y=w268) -> (max(x,y)=w270:dbl)  [unwired: 1 out]
    "Max top" <- w270
    n136 = feedback-in #2(w270) -> ()
    n137 = shared-variable ".\\Untitled Library 1.lvlib\\Rpm2"(w246) -> ()  [unwired: 1 in, 1 out]
    n138 = Bundle("Top Cntrl"="Top Cntrl", w246) -> ()  [unwired: 1 in, 1 out]
    n139 = shared-variable ".\\Untitled Library 1.lvlib\\Control Signal2"(w271) -> ()  [unwired: 1 in, 1 out]
    n140 = feedback #3(w261) -> (w264:dbl)
    n141 = Select(t=inf, s="reset top", f=w264) -> (s? t:f=w266:dbl)
    n142 = Max & Min(x=w246, y=w266) -> (min(x,y)=w265:dbl)  [unwired: 1 out]
    "Min Top" <- w265
    n143 = feedback-in #3(w265) -> ()
    n144 = Add(x="Top Cntrl", y="Top Tol") -> (x+y=w276:dbl)
    n145 = Subtract(x="Top Cntrl", y="Top Tol") -> (x-y=w275:dbl)
    n146 = Subtract(x="Top Cntrl", y=w246) -> (x-y=w296:dbl)
    n147 = Less Than 0?(x=w296) -> (x < 0?=→"RPM High":bool)
    n148 = Greater Than 0?(x=w296) -> (x > 0?=→"RPM Low":bool)
    n149 = Absolute Value(x=w296) -> (abs(x)=w293:dbl)
    n150 = In Range and Coerce(upper limit=w276, x=w246, lower limit=w275) -> (In Range?=→"RPM Steady? Top":bool)  [unwired: 1 out]
    n151 = Less Or Equal?(x=w293, y=1.0) -> (x <= y?=→"1 RPM":bool)
    n152 = Less Or Equal?(x=w293, y=2.0) -> (x <= y?=→"2 RPM":bool)
    n153 = Less Or Equal?(x=w293, y=3.0) -> (x <= y?=→"3 RPM":bool)
    n154 = Less Or Equal?(x=w293, y=4.0) -> (x <= y?=→"4 RPM":bool)
    n155 = Less Or Equal?(x=w293, y=5.0) -> (x <= y?=→"5 RPM":bool)
    n156 = Less Or Equal?(x=w293, y=6.0) -> (x <= y?=→"6 RPM":bool)
    n157 = Less Or Equal?(x=w293, y=7.0) -> (x <= y?=→"7 RPM":bool)
    n158 = Less Or Equal?(x=w293, y=8.0) -> (x <= y?=→"8 RPM":bool)
    n159 = feedback #4(0) -> (w252:i32)
    "State1" <- w252
    n160 = feedback #5(w252) -> (w251:i32)
    n161 = feedback-in #5(w252) -> ()
    n162 = case shown="0, Default" w252 {
      selector: w252 -> [w309 w344 _]
      tunnel: w246 -> [w315 w335 w353]
      tunnel: [w331 w339 w352] -> w249
      tunnel: "Arm" -> [w330 _ _]
      tunnel: "Trig" -> [w311 _ _]
      tunnel: w251 -> [w310 w343 _]
      tunnel: "Len" -> [_ w341 _]
      tunnel: [w315 w335 w353] -> w256
      tunnel: "Reset1" -> [w307 _ w349]
      tunnel: [TRUE TRUE FALSE] -> w255
      frame 0, Default {
        w329 = 0
        n163 = Less?(x=w309, y=w310) -> (x < y?=w308:bool)
        n164 = Or(x=w307, y=w308) -> (x .or. y?=w306:bool)
        n165 = feedback #6(-inf) -> (w321:dbl)
        n166 = Select(t=w315, s=w306, f=w321) -> (s? t:f=w320:dbl)
        n167 = Max & Min(x=w315, y=w320) -> (max(x,y)=w327:dbl)  [unwired: 1 out]
        n168 = feedback-in #6(w327) -> ()
        n169 = feedback #7(inf) -> (w319:dbl)
        n170 = Select(t=w315, s=w306, f=w319) -> (s? t:f=w318:dbl)
        n171 = Max & Min(x=w315, y=w318) -> (min(x,y)=w326:dbl)  [unwired: 1 out]
        n172 = Add(x=w326, y=w327) -> (x+y=w325:dbl)
        n173 = Divide(x=w325, y=2.0) -> (x/y=w314:dbl)
        n174 = feedback-in #7(w326) -> ()
        n175 = Add(x=w311, y=w314) -> (x+y=w317:dbl)
        n176 = Subtract(x=w314, y=w311) -> (x-y=w316:dbl)
        n177 = In Range and Coerce(upper limit=w317, x=w315, lower limit=w316) -> (In Range?=w313:bool)  [unwired: 1 out]
        n178 = Not(x=w313) -> (.not. x?=w312:bool)
        "Tgrd" <- w312
        n179 = Select(t=1, s=w312, f=w329) -> (s? t:f=w332:i32)
        n180 = Select(t=w332, s=w330, f=w329) -> (s? t:f=w331:i32)
      }
      frame 1 {
        w346 = i16 0
        n181 = Greater?(x=w344, y=w343) -> (0:w342:bool)
        n182 = feedback #8(w346) -> (w347:i16)
        n183 = Select(t=w346, s=w342, f=w347) -> (s? t:f=w345:i16)
        n184 = Increment(x=w345) -> (x+1=w340:i16)
        "cnt" <- w340
        n185 = feedback-in #8(w340) -> ()
        n186 = Greater Or Equal?(x=w340, y=w341) -> (x >= y?=w336:bool)
        n187 = Select(t=2, s=w336, f=1) -> (s? t:f=w339:i32)
      }
      frame 2 {
        n188 = Select(t=0, s=w349, f=2) -> (s? t:f=w352:i32)
      }
    }
    n189 = feedback-in #4(w249) -> ()
    n190 = case shown="True" w255 {
      tunnel: w256 -> [_ w305]
      tunnel: "Top Cntrl" -> [_ w303]
      frame False {
      }
      frame True {
        n191 = Bundle(w305, "Top Cntrl"=w303) -> (→"Top Response":cluster{dbl, "Top Cntrl":dbl})  [unwired: 1 in]
      }
    }
    n192 = node-c288("Top Period") -> ()  [unwired: 1 in, 1 out]
    "Top Cntrl ." <- "Top Cntrl"
  }
  n193 = call <vilib>:"WPI_EncoderRefNum Registry Get.vi"("refnum name"="BottomWheelSpeed") -> ("EncoderDevRef"=w52:T17)  [unwired: 9 in, 1 out]
  n194 = call <vilib>:"WPI_MotorControlRefNum Registry Get.vi"("refnum name"="BottomMotor") -> ("MotorControlDevRef"=w51:T13)  [unwired: 9 in, 1 out]
  n195 = node-c288(w5) -> ()  [unwired: 1 out]
  n196 = node-c288() -> (w8:T8)  [unwired: 4 in]
  n197 = timed-loop {
    timing: w8 -> [_]
    timing-out: [_] -> w7
    tunnel: w52 -> [w474]
    tunnel: w51 -> [w476]
    i -> [w442]
    stop <- FALSE stop-if-true
    w433 = -inf
    w432 = inf
    n198 = node-c288() -> (→"Bot Late?":bool)  [unwired: 1 in, 1 out]
    n199 = case shown="True" TRUE {
      tunnel: w476 -> [w537 w597]
      tunnel: w474 -> [_ _]
      tunnel: "BotInvert" -> [w561 _]
      tunnel: "Bot Cntrl" -> [w530 w581]
      tunnel: "Disable Bottom" -> [w557 _]
      tunnel: "Open?" -> [w556 w580]
      tunnel: "Open Loop Cntrl" -> [w555 w579]
      tunnel: [w532 w586] -> w443
      tunnel: w442 -> [w546 _]
      tunnel: [w529 w578] -> w418
      tunnel: [w530 w581] -> w417
      tunnel: [w538 w582] -> w430
      frame False {
        n200 = call <vilib>:"WPI_CANTalonSRX_GetStatus.vi"("CAN Talon SRX Ref"=w537) -> ("Talon SRX Status"=w540:T23)  [unwired: 8 in, 2 out]
        n201 = Unbundle By Name(w540) -> ("Encoder Velocity"=w539:dbl, "Encoder Position"=w538:dbl)
        n202 = Quotient & Remainder(x=w546, y=2) -> (x-y*floor(x/y)=w548:i32)  [unwired: 1 out]
        n203 = Equal To 0?(x=w548) -> (x = 0?=w547:bool)
        n204 = call <userlib>:"UpDown_Counter.vi"("up"=w547) -> ("count"=w545:i32)  [unwired: 4 in]
        "Iter" <- w545
        n205 = Divide(x="Enc Counts 3", y=600.0) -> (x/y=w541:dbl)
        n206 = Negate(x=w539) -> (-x=w534:dbl)
        n207 = Divide(x=w534, y=w541) -> (x/y=w529:dbl)
        n208 = Equal To 0?(x="Bot tbh Gain") -> (x = 0?=w533:bool)
        n209 = call "tbhwithreinitialize.vi"("Gain"="Bot tbh Gain", "Act"=w529, "Cmd"=w530) -> ("Out"=w528:dbl)
        n210 = Select(t="Bot tbh Gain", s=w533, f=w528) -> (s? t:f=w532:dbl)
        n211 = feedback #9(FALSE) -> (w551:bool)
        "State" <- w551
        n212 = case shown="True" w551 {
          tunnel: [0.5 w572] -> w553
          tunnel: w532 -> [_ w573]
          tunnel: [w564 w576] -> w552
          tunnel: w545 -> [w563 w574]
          tunnel: "delay" -> [w562 w575]
          tunnel: w530 -> [_ w568]
          frame False {
            n213 = Greater Or Equal?(x=w563, y=w562) -> (x >= y?=w564:bool)
          }
          frame True {
            n214 = Multiply(x=w568, y="FF Gain") -> (x*y=w567:dbl)
            n215 = Select(t=w567, s="FF", f=0.0) -> (s? t:f=w571:dbl)
            n216 = Add(x=w573, y=w571) -> (x+y=w572:dbl)
            n217 = Greater Or Equal?(x=w574, y=w575) -> (x >= y?=w576:bool)
          }
        }
        n218 = Negate(x=w553) -> (-x=w560:dbl)
        n219 = Select(t=w560, s=w561, f=w553) -> (s? t:f=w559:dbl)
        n220 = Select(t=w555, s=w556, f=w559) -> (s? t:f=w558:dbl)
        n221 = Select(t=0.0, s=w557, f=w558) -> (s? t:f=w536:dbl)
        n222 = call <vilib>:"WPI_CANTalonSRX_ChangeMode.vi"("Output"=w536, "Control Mode"=WPI_CANTalonSRX_APIControlMode."Percent VBus", "CAN Talon SRX Ref"=w537) -> ()  [unwired: 7 in, 2 out]
        n223 = feedback-in #9(w552) -> ()
      }
      frame True {
        n224 = call <vilib>:"WPI_CANTalonSRX_SetReference.vi"("Reverse Feedback Sensor"="Rev FB Sensor", "Feedback Reference"=WPI_CANTalonSRX_APIFeedbackSelect."Digital Quadrature Encoder", "CAN Talon SRX Ref"=w597) -> ("CAN Talon SRX Ref"=w601:T13)  [unwired: 7 in, 1 out]
        n225 = Divide(x="Enc Counts", y=600.0) -> (x/y=w589:dbl)
        n226 = Multiply(x=w589, y=w581) -> (x*y=w585:dbl)
        n227 = call <vilib>:"WPI_CANTalonSRX_SetPID.vi"("CAN Talon SRX Ref"=w601, "P"="P 3", "I"="I 3", "D"="D 3", "F"="F 3", "I Zone"="I Zone 3", "Ramp Rate"="Ramp Rate 3") -> ("CAN Talon SRX Ref"=w603:T13)  [unwired: 7 in, 1 out]
        n228 = Negate(x=w585) -> (-x=w584:dbl)
        n229 = case shown="True" w580 {
          tunnel: w603 -> [w607 w611]
          tunnel: [w606 w610] -> w602
          tunnel: w584 -> [_ w608]
          tunnel: w579 -> [w604 _]
          frame True {
            n230 = call <vilib>:"WPI_CANTalonSRX_ChangeMode.vi"("Output"=w604, "Control Mode"=WPI_CANTalonSRX_APIControlMode."Percent VBus", "CAN Talon SRX Ref"=w607) -> ("CAN Talon SRX Ref"=w606:T13)  [unwired: 7 in, 1 out]
          }
          frame False {
            n231 = call <vilib>:"WPI_CANTalonSRX_ChangeMode.vi"("Output"=w608, "Control Mode"=WPI_CANTalonSRX_APIControlMode."Speed", "CAN Talon SRX Ref"=w611) -> ("CAN Talon SRX Ref"=w610:T13)  [unwired: 7 in, 1 out]
          }
        }
        n232 = disable-structure shown="Disabled" {
          frame Disabled {
            n233 = call "RPM2FF.vi"() -> ()  [unwired: 11 in, 1 out]
          }
          frame Enabled {
          }
        }
        n234 = call <vilib>:"WPI_CANTalonSRX_GetStatus.vi"("CAN Talon SRX Ref"=w602) -> ("Talon SRX Status"=w600:T23)  [unwired: 8 in, 2 out]
        n235 = Unbundle By Name(w600) -> ("Encoder Velocity"=w588:dbl, "Applied Throttle"=w586:dbl, "Encoder Position"=w582:dbl)
        n236 = Negate(x=w588) -> (-x=w583:dbl)
        n237 = Divide(x=w583, y=w589) -> (x/y=w587:dbl)
        n238 = Negate(x=w587) -> (-x=w578:dbl)
      }
    }
    "Bot Cntrl ." <- w417
    "Bot Dist" <- w430
    n239 = case shown="True" "Log Bot Current?" {
      frame False {
      }
      frame True {
        n240 = call <vilib>:"WPI_Power Get PDP Currents.vi"("PDP Channel"="Bot Channel") -> ("current (A)"=w614:dbl)  [unwired: 12 in, 2 out]
        "Bot Current" <- w614
        n241 = shared-variable ".\\Untitled Library 1.lvlib\\Current1"(w614) -> ()  [unwired: 1 in, 1 out]
        n242 = call <vilib>:"WPI_Power Get PDP Currents.vi"("PDP Channel"="Bot Channel 2") -> ("current (A)"=w613:dbl)  [unwired: 12 in, 2 out]
        "Bot Current 2" <- w613
        n243 = shared-variable ".\\Untitled Library 1.lvlib\\Current3"(w613) -> ()  [unwired: 1 in, 1 out]
      }
    }
    n244 = Bundle("Bot Cntrl"=w417, w418) -> ()  [unwired: 1 in, 1 out]
    n245 = Add(x=w417, y="Bot Tol") -> (x+y=w467:dbl)
    n246 = Subtract(x=w417, y="Bot Tol") -> (x-y=w468:dbl)
    n247 = feedback #10(w433) -> (w439:dbl)
    n248 = Select(t=w433, s="reset bot", f=w439) -> (s? t:f=w438:dbl)
    n249 = shared-variable ".\\Untitled Library 1.lvlib\\Rpm1"(w418) -> ()  [unwired: 1 in, 1 out]
    n250 = shared-variable ".\\Untitled Library 1.lvlib\\Control Signal1"(w443) -> ()  [unwired: 1 in, 1 out]
    n251 = Subtract(x=w417, y=w418) -> (x-y=w447:dbl)
    n252 = Max & Min(x=w418, y=w438) -> (max(x,y)=w440:dbl)  [unwired: 1 out]
    "Max Bot" <- w440
    n253 = feedback-in #10(w440) -> ()
    n254 = Less Than 0?(x=w447) -> (x < 0?=→"RPM High .":bool)
    n255 = Greater Than 0?(x=w447) -> (x > 0?=→"RPM Low .":bool)
    n256 = Absolute Value(x=w447) -> (abs(x)=w450:dbl)
    n257 = In Range and Coerce(upper limit=w467, x=w418, lower limit=w468) -> (In Range?=→"RPM Steady? 2":bool)  [unwired: 1 out]
    n258 = feedback #11(w432) -> (w434:dbl)
    n259 = Select(t=w432, s="reset bot", f=w434) -> (s? t:f=w437:dbl)
    n260 = Max & Min(x=w418, y=w437) -> (min(x,y)=w435:dbl)  [unwired: 1 out]
    "Min Bot" <- w435
    n261 = feedback-in #11(w435) -> ()
    n262 = Less Or Equal?(x=w450, y=1.0) -> (x <= y?=→"1 RPM .":bool)
    n263 = Less Or Equal?(x=w450, y=2.0) -> (x <= y?=→"2 RPM .":bool)
    n264 = Less Or Equal?(x=w450, y=3.0) -> (x <= y?=→"3 RPM .":bool)
    n265 = Less Or Equal?(x=w450, y=4.0) -> (x <= y?=→"4 RPM .":bool)
    n266 = Less Or Equal?(x=w450, y=5.0) -> (x <= y?=→"5 RPM .":bool)
    n267 = Less Or Equal?(x=w450, y=6.0) -> (x <= y?=→"6 RPM .":bool)
    n268 = Less Or Equal?(x=w450, y=7.0) -> (x <= y?=→"7 RPM .":bool)
    n269 = Less Or Equal?(x=w450, y=8.0) -> (x <= y?=→"8 RPM .":bool)
    n270 = feedback #12(0) -> (w424:i32)
    "State2" <- w424
    n271 = feedback #13(w424) -> (w423:i32)
    n272 = feedback-in #13(w424) -> ()
    n273 = case shown="0, Default" w424 {
      selector: w424 -> [w483 w518 _]
      tunnel: w418 -> [w489 w509 w527]
      tunnel: [w505 w513 w526] -> w421
      tunnel: "Arm2" -> [w504 _ _]
      tunnel: "Trig2" -> [w485 _ _]
      tunnel: w423 -> [w484 w517 _]
      tunnel: "Len2" -> [_ w515 _]
      tunnel: [w489 w509 w527] -> w428
      tunnel: "Reset2" -> [w481 _ w523]
      tunnel: [TRUE TRUE FALSE] -> w427
      frame 0, Default {
        w503 = 0
        n274 = Less?(x=w483, y=w484) -> (x < y?=w482:bool)
        n275 = Or(x=w481, y=w482) -> (x .or. y?=w480:bool)
        n276 = feedback #14(-inf) -> (w495:dbl)
        n277 = Select(t=w489, s=w480, f=w495) -> (s? t:f=w494:dbl)
        n278 = Max & Min(x=w489, y=w494) -> (max(x,y)=w501:dbl)  [unwired: 1 out]
        n279 = feedback-in #14(w501) -> ()
        n280 = feedback #15(inf) -> (w493:dbl)
        n281 = Select(t=w489, s=w480, f=w493) -> (s? t:f=w492:dbl)
        n282 = Max & Min(x=w489, y=w492) -> (min(x,y)=w500:dbl)  [unwired: 1 out]
        n283 = Add(x=w500, y=w501) -> (x+y=w499:dbl)
        n284 = Divide(x=w499, y=2.0) -> (x/y=w488:dbl)
        n285 = feedback-in #15(w500) -> ()
        n286 = Add(x=w485, y=w488) -> (x+y=w491:dbl)
        n287 = Subtract(x=w488, y=w485) -> (x-y=w490:dbl)
        n288 = In Range and Coerce(upper limit=w491, x=w489, lower limit=w490) -> (In Range?=w487:bool)  [unwired: 1 out]
        n289 = Not(x=w487) -> (.not. x?=w486:bool)
        "Tgrd 2" <- w486
        n290 = Select(t=1, s=w486, f=w503) -> (s? t:f=w506:i32)
        n291 = Select(t=w506, s=w504, f=w503) -> (s? t:f=w505:i32)
      }
      frame 1 {
        w520 = i16 0
        n292 = Greater?(x=w518, y=w517) -> (0:w516:bool)
        n293 = feedback #16(w520) -> (w521:i16)
        n294 = Select(t=w520, s=w516, f=w521) -> (s? t:f=w519:i16)
        n295 = Increment(x=w519) -> (x+1=w514:i16)
        "cnt 2" <- w514
        n296 = feedback-in #16(w514) -> ()
        n297 = Greater Or Equal?(x=w514, y=w515) -> (x >= y?=w510:bool)
        n298 = Select(t=2, s=w510, f=1) -> (s? t:f=w513:i32)
      }
      frame 2 {
        n299 = Select(t=0, s=w523, f=2) -> (s? t:f=w526:i32)
      }
    }
    n300 = feedback-in #12(w421) -> ()
    n301 = case shown="True" w427 {
      tunnel: w428 -> [_ w479]
      tunnel: w417 -> [_ w478]
      frame False {
      }
      frame True {
        n302 = Bundle(w479, "Bot Cntrl"=w478) -> (→"Bot Response":cluster{dbl, "Bot Cntrl":dbl})  [unwired: 1 in]
      }
    }
    n303 = node-c288("Bot Period") -> ()  [unwired: 1 in, 1 out]
  }
  n304 = call <vilib>:"WPI_JoystickRefNum Registry Get.vi"("refnum name"="Joystick") -> ("JoystickDevRef"=w34:T24)  [unwired: 9 in, 1 out]
  n305 = node-c288(w7) -> ()  [unwired: 1 out]
  n306 = call <vilib>:"WPI_DigitalInputOpen.vi"("DIO Channel"=FPGA_DIOChannel."DIO 4") -> ("DigitalInputDevRef"=w11:T26)  [unwired: 9 in, 1 out]
  n307 = call <vilib>:"WPI_DigitalInputOpen.vi"("DIO Channel"=FPGA_DIOChannel."DIO 5") -> ("DigitalInputDevRef"=w10:T26)  [unwired: 9 in, 1 out]
  n308 = call <vilib>:"WPI_MotorControlRefNum Registry Get.vi"("refnum name"="TurretMotor") -> ("MotorControlDevRef"=w16:T13)  [unwired: 9 in, 1 out]
  n309 = node-c288(i64 20 ("Period")) -> (w18:T8)  [unwired: 3 in]
  n310 = timed-loop {
    timing: w18 -> [_]
    timing-out: [_] -> w17
    tunnel: w16 -> [w637]
    tunnel: w34 -> [w624]
    tunnel: w11 -> [w636]
    tunnel: w10 -> [w635]
    border: 0.0 -> [_]
    stop <- FALSE stop-if-true
    # "Turret Control"
    n311 = node-c288() -> (→"TurretLate?":bool)  [unwired: 1 in]
    n312 = shared-variable ".\\MaddenSharedVariables.lvlib\\Turret Yaw"() -> (w628:dbl)  [unwired: 1 in, 1 out]
    n313 = shared-variable ".\\MaddenSharedVariables.lvlib\\Robot Yaw"() -> (w627:dbl)  [unwired: 1 in, 1 out]
    n314 = call <vilib>:"WPI_DigitalInputGetValue.vi"("DigitalInputDevRef"=w636) -> ("Value"=w634:bool)  [unwired: 8 in, 2 out]
    n315 = call <vilib>:"WPI_DigitalInputGetValue.vi"("DigitalInputDevRef"=w635) -> ("Value"=w633:bool)  [unwired: 8 in, 2 out]
    n316 = Not(x=w633) -> (.not. x?=w625:bool)
    n317 = Not(x=w634) -> (.not. x?=w623:bool)
    n318 = Subtract(x=w627, y=w628) -> (x-y=w631:dbl)
    n319 = Or(x=w625, y=w623) -> (x .or. y?=w632:bool)
    n320 = feedback #17() -> (w629:dbl)
    n321 = case shown="True" w632 {
      tunnel: w625 -> [_ w764]
      tunnel: w631 -> [_ w765]
      tunnel: [w759 w760] -> w630
      tunnel: w629 -> [w759 _]
      frame False {
      }
      frame True {
        n322 = Negate(x="Out Bound") -> (-x=w762:dbl)
        n323 = Select(t=w762, s=w764, f="Out Bound") -> (s? t:f=w761:dbl)
        n324 = Subtract(x=w761, y=w765) -> (x-y=w760:dbl)
      }
    }
    n325 = feedback-in #17(w630) -> ()
    n326 = Add(x=w631, y=w629) -> (x+y=w626:dbl)
    n327 = case shown="True" TRUE {
      tunnel: w637 -> [_ w709]
      tunnel: w626 -> [_ w663]
      tunnel: w625 -> [_ w695]
      tunnel: w624 -> [w640 w693]
      tunnel: w623 -> [_ w696]
      frame False {
        n328 = call <vilib>:"WPI_JoystickGetValues.vi"("JoystickDevRef"=w640) -> ("Buttons"=w639:bool[])  [unwired: 6 in, 4 out]
        n329 = Index Array(array=w639, index #1=4 ("index"), index #2=5 ("index")) -> (element #1=w643:bool, element #2=w644:bool)
        n330 = Select(t=-1.0, s=w643, f=0.0) -> (s? t:f=w646:dbl)
        n331 = Select(t=1.0, s=w644, f=w646) -> ()  [unwired: 1 out]
        n332 = case shown="True" "SoftStop" {
          tunnel: [0.0 ("Motor Out") w651] -> _
          frame False {
          }
          frame True {
            n333 = shared-variable ".\\MaddenSharedVariables.lvlib\\Robot Yaw"() -> ()  [unwired: 1 in, 2 out]
            n334 = shared-variable ".\\MaddenSharedVariables.lvlib\\Turret Yaw"() -> (w654:dbl)  [unwired: 1 in, 1 out]
            n335 = Subtract(x=w654, y=0.0) -> (x-y=w653:dbl)
            "Angle" <- w653
            n336 = call <userlib>:"Soft_Stops.vi"("correlation"="correlation", "Sense"=w653, "Lo Limit"="Lo Limit", "Hi Limit"="Hi Limit", "Speed near Limit"="Speed near Limit", "Near Limit"="Near Limit") -> ("Motor Out"=w651:dbl, "At Lo"=→"At Lo":bool, "At Hi"=→"At Hi":bool)  [unwired: 7 in]
            "Motor Out" <- w651
          }
        }
      }
      frame True {
        n337 = call <vilib>:"WPI_JoystickGetValues.vi"("JoystickDevRef"=w693) -> ("Buttons"=w685:bool[])  [unwired: 6 in, 4 out]
        n338 = shared-variable ".\\MaddenSharedVariables.lvlib\\Boiler Valid"() -> (w679:bool)  [unwired: 1 in, 1 out]
        n339 = shared-variable ".\\MaddenSharedVariables.lvlib\\Boiler Yaw"() -> (w677:dbl)  [unwired: 1 in, 1 out]
        n340 = Index Array(array=w685, index #1=4 ("index"), index #2=5 ("index")) -> (element #1=w684:bool, element #2=w688:bool)
        n341 = Add(x=w663, y=w677) -> (x+y=w700:dbl)
        n342 = Select(t=w700, s=w679, f=w663) -> (s? t:f=w699:dbl)
        n343 = Select(t=w699, s="Track Target", f="desired Angle") -> (s? t:f=w703:dbl)
        n344 = Select(t=-1.0, s=w684, f=0.0) -> (s? t:f=w690:dbl)
        n345 = Absolute Value(x=w677) -> (abs(x)=w673:dbl)
        n346 = Select(t=1.0, s=w688, f=w690) -> (s? t:f=w682:dbl)
        n347 = Less?(x=w673, y="Tolerance") -> (x < y?=w675:bool)
        n348 = Multiply(x="Turret Max Speed", y=w682) -> (x*y=w681:dbl)
        n349 = feedback #18(0) -> (w667:i32)
        "State1 2" <- w667
        n350 = feedback #19(w667) -> (w668:i32)
        n351 = feedback-in #19(w667) -> ()
        n352 = case shown="0, Default" w667 {
          selector: w667 -> [w714 w749 _]
          tunnel: w663 -> [w720 w740 w758]
          tunnel: [w736 w744 w757] -> w670
          tunnel: "Arm 2" -> [w735 _ _]
          tunnel: "Trig 2" -> [w716 _ _]
          tunnel: w668 -> [w715 w748 _]
          tunnel: "Len 2" -> [_ w746 _]
          tunnel: [w720 w740 w758] -> w662
          tunnel: "Reset1 2" -> [w712 _ w754]
          tunnel: [TRUE TRUE FALSE] -> w664
          frame 0, Default {
            w734 = 0
            n353 = Less?(x=w714, y=w715) -> (x < y?=w713:bool)
            n354 = Or(x=w712, y=w713) -> (x .or. y?=w711:bool)
            n355 = feedback #20(-inf) -> (w726:dbl)
            n356 = Select(t=w720, s=w711, f=w726) -> (s? t:f=w725:dbl)
            n357 = Max & Min(x=w720, y=w725) -> (max(x,y)=w732:dbl)  [unwired: 1 out]
            n358 = feedback-in #20(w732) -> ()
            n359 = feedback #21(inf) -> (w724:dbl)
            n360 = Select(t=w720, s=w711, f=w724) -> (s? t:f=w723:dbl)
            n361 = Max & Min(x=w720, y=w723) -> (min(x,y)=w731:dbl)  [unwired: 1 out]
            n362 = Add(x=w731, y=w732) -> (x+y=w730:dbl)
            n363 = Divide(x=w730, y=2.0) -> (x/y=w719:dbl)
            n364 = feedback-in #21(w731) -> ()
            n365 = Add(x=w716, y=w719) -> (x+y=w722:dbl)
            n366 = Subtract(x=w719, y=w716) -> (x-y=w721:dbl)
            n367 = In Range and Coerce(upper limit=w722, x=w720, lower limit=w721) -> (In Range?=w718:bool)  [unwired: 1 out]
            n368 = Not(x=w718) -> (.not. x?=w717:bool)
            "Tgrd 3" <- w717
            n369 = Select(t=1, s=w717, f=w734) -> (s? t:f=w737:i32)
            n370 = Select(t=w737, s=w735, f=w734) -> (s? t:f=w736:i32)
          }
          frame 1 {
            w751 = i16 0
            n371 = Greater?(x=w749, y=w748) -> (0:w747:bool)
            n372 = feedback #22(w751) -> (w752:i16)
            n373 = Select(t=w751, s=w747, f=w752) -> (s? t:f=w750:i16)
            n374 = Increment(x=w750) -> (x+1=w745:i16)
            "cnt 3" <- w745
            n375 = feedback-in #22(w745) -> ()
            n376 = Greater Or Equal?(x=w745, y=w746) -> (x >= y?=w741:bool)
            n377 = Select(t=2, s=w741, f=1) -> (s? t:f=w744:i32)
          }
          frame 2 {
            n378 = Select(t=0, s=w754, f=2) -> (s? t:f=w757:i32)
          }
        }
        n379 = feedback-in #18(w670) -> ()
        n380 = Bundle(w662, "desired Angle"=w703) -> (w704:cluster{dbl, "desired Angle":dbl})  [unwired: 1 in]
        n381 = Not(x=w679) -> (.not. x?=w678:bool)
        n382 = Or(x=w675, y=w678) -> (x .or. y?=w674:bool)
        n383 = call "Turret-firstVI.vi"("MotorControlDevRef"=w709, "PID gains"="PID gains", "Soft Stops"="Soft Stops", "Joystick Input"=w681, "output range"="output range", "Positive soft stop"=w695, "reinitialize? (F)"=w674, "Negative soft stop"=w696, "shooter range"="shooter range", "Manual"="Manual", "Current angle"=w663, "Eval Period Soft Stops"="Soft Stop Period", "desired Angle"=w703, "Softstop"="Softstop") -> ("Motor Output"=→"Motor Output":dbl)  [unwired: 1 in]
        n384 = case shown="True" w664 {
          tunnel: w704 -> [_ w710]
          frame False {
          }
          frame True {
            "Turret" <- w710
          }
        }
        "TtR" <- w663
      }
    }
    n385 = node-c288() -> ()  [unwired: 1 in, 1 out]
  }
  n386 = call <vilib>:"WPI_MotorControlRefNum Registry Get.vi"("refnum name"="IntakeMotor") -> ("MotorControlDevRef"=w36:T13)  [unwired: 9 in, 1 out]
  n387 = call <vilib>:"WPI_MotorControlRefNum Registry Get.vi"("refnum name"="AgitatorMotor") -> ("MotorControlDevRef"=w28:T13)  [unwired: 9 in, 1 out]
  n388 = call <vilib>:"WPI_MotorControlRefNum Registry Get.vi"("refnum name"="PrimerMotor") -> ("MotorControlDevRef"=w27:T13)  [unwired: 9 in, 1 out]
  n389 = node-c288(i64 50 ("Period")) -> (w40:T8)  [unwired: 3 in]
  n390 = timed-loop {
    timing: w40 -> [_]
    timing-out: [_] -> w39
    tunnel: w34 -> [w783]
    tunnel: w36 -> [w770]
    stop <- FALSE stop-if-true
    # "Intake Test Loop"
    n391 = node-c288() -> ()  [unwired: 1 in, 1 out]
    n392 = call <vilib>:"WPI_JoystickGetValues.vi"("JoystickDevRef"=w783) -> ("JoystickDevRef"=w782:T24)  [unwired: 6 in, 4 out]
    n393 = call <vilib>:"WPI_JoystickGetValues.vi"("JoystickDevRef"=w782) -> ("Buttons"=w781:bool[])  [unwired: 6 in, 4 out]
    n394 = Index Array(array=w781, index=0) -> (element=w779:bool)
    n395 = Select(t=1.0, s=w779, f=0.0) -> (s? t:f=w776:dbl)
    n396 = Multiply(x=w776, y="Intake Speed") -> (x*y=w772:dbl)
    n397 = Negate(x=w772) -> (-x=w773:dbl)
    n398 = Select(t=w773, s="Invert Intake", f=w772) -> (s? t:f=w771:dbl)
    n399 = call <vilib>:"WPI_MotorControlSetOutput.vi"("Output"=w771, "MotorControlDevRef"=w770) -> ()  [unwired: 7 in, 3 out]
    n400 = node-c288() -> ()  [unwired: 1 in, 1 out]
  }
  n401 = node-c288(i64 50 ("Period")) -> (w33:T8)  [unwired: 3 in]
  n402 = timed-loop {
    timing: w33 -> [_]
    timing-out: [_] -> w32
    tunnel: w28 -> [w802]
    tunnel: w27 -> [w790]
    tunnel: w34 -> [w810]
    stop <- FALSE stop-if-true
    # "FMS Loop"
    n403 = node-c288() -> ()  [unwired: 1 in, 1 out]
    n404 = call <vilib>:"WPI_JoystickGetValues.vi"("JoystickDevRef"=w810) -> ("Buttons"=w809:bool[])  [unwired: 6 in, 4 out]
    n405 = Index Array(array=w809, index #1=6 ("index"), index #2=7 ("index")) -> (element #1=w805:bool, element #2=w806:bool)
    n406 = Or(x=w805, y=w806) -> (x .or. y?=w791:bool)
    n407 = Multiply(x="Agitator Max Speed", y=1.0) -> (x*y=w801:dbl)
    n408 = Multiply(x="Primer Max Speed", y=1.0) -> (x*y=w793:dbl)
    n409 = Negate(x=w801) -> (-x=w803:dbl)
    n410 = Negate(x=w793) -> (-x=w792:dbl)
    n411 = Select(t=w803, s="Invert Agitator", f=w801) -> (s? t:f=w797:dbl)
    n412 = Select(t=w792, s="Invert Primer", f=w793) -> (s? t:f=w789:dbl)
    n413 = Select(t=w797, s=w791, f=0.0) -> (s? t:f=w796:dbl)
    n414 = Select(t=w789, s=w791, f=0.0) -> (s? t:f=w795:dbl)
    n415 = call <vilib>:"WPI_MotorControlSetOutput.vi"("Output"=w796, "MotorControlDevRef"=w802) -> ()  [unwired: 7 in, 3 out]
    n416 = call <vilib>:"WPI_MotorControlSetOutput.vi"("Output"=w795, "MotorControlDevRef"=w790) -> ()  [unwired: 7 in, 3 out]
    n417 = node-c288() -> ()  [unwired: 1 in, 1 out]
  }
  n418 = call <userlib>:"IMUOrientRefNum_Registry_Get.vi"("refnum name"="Pri IMU") -> ("I2CDevRef out"=w44:T27)  [unwired: 9 in, 1 out]
  n419 = call <userlib>:"IMUOrientRefNum_Registry_Get.vi"("refnum name"="Alt IMU") -> ("I2CDevRef out"=w41:T27)  [unwired: 9 in, 1 out]
  n420 = node-c288(i64 20 ("Period")) -> (w47:T8)  [unwired: 3 in]
  n421 = timed-loop {
    timing: w47 -> [_]
    timing-out: [_] -> w46
    tunnel: w44 -> [w823]
    tunnel: w41 -> [w816]
    stop <- FALSE stop-if-true
    n422 = node-c288() -> ()  [unwired: 1 in, 1 out]
    n423 = call <userlib>:"IMUOrientRead.vi"("I2CDevRef"=w816) -> ("Orient Y/R/P"=w817:T29)  [unwired: 8 in, 6 out]
    n424 = call <userlib>:"IMUOrientRead.vi"("I2CDevRef"=w823) -> ("Orient Y/R/P"=w822:T29)  [unwired: 8 in, 6 out]
    n425 = Unbundle By Name(w817) -> ("Yaw Wind"=w815:dbl, "Roll"=w818:dbl, "Pitch"=w819:dbl)
    n426 = Unbundle By Name(w822) -> ("Yaw Wind"=w814:dbl, "Roll"=w821:dbl, "Pitch"=w820:dbl)
    n427 = disable-structure shown="Disabled" {
      disable-tunnel: w819 -> [w827 _]
      disable-tunnel: w818 -> [w826 _]
      disable-tunnel: w815 -> [w825 _]
      frame Disabled {
        "Roll Alt" <- w826
        "Pitch Alt" <- w827
        "Yaw Alt" <- w825
      }
      frame Enabled {
      }
    }
    n428 = disable-structure shown="Disabled" {
      disable-tunnel: w821 -> [w830 _]
      disable-tunnel: w820 -> [w829 _]
      disable-tunnel: w814 -> [w828 _]
      frame Disabled {
        "Roll" <- w830
        "Pitch" <- w829
        "Yaw" <- w828
      }
      frame Enabled {
      }
    }
    n429 = shared-variable ".\\MaddenSharedVariables.lvlib\\Turret Yaw"(w814) -> ()  [unwired: 1 in, 1 out]
    n430 = shared-variable ".\\MaddenSharedVariables.lvlib\\Robot Yaw"(w815) -> ()  [unwired: 1 in, 1 out]
    n431 = node-c288() -> ()  [unwired: 1 in, 1 out]
  }
  n432 = node-c288(w32) -> ()  [unwired: 1 out]
  n433 = node-c288(w39) -> ()  [unwired: 1 out]
  n434 = node-c288(w17) -> ()  [unwired: 1 out]
  n435 = node-c288(w46) -> ()  [unwired: 1 out]
  n436 = call <vilib>:"WPI_RobotDriveRefNum Registry Get.vi"("refnum name"="Drive Motors") -> ("RobotDriveDevRef"=w24:T30)  [unwired: 9 in, 1 out]
  n437 = call <userlib>:"Drive_Loop_Initialize.vi"("Name of drive loop (give it a name!)"="Drive Loop") -> ("Drive Loop Cluster"=w21:T31)  [unwired: 9 in, 1 out]
  n438 = call <userlib>:"Drive_Loop_Control_Loop.vi"("Period \n- Amount of time between iterations of the timed control loop"=i64 50 ("Period \n- Amount of time between iterations of the timed control loop"), "RobotDriveDevRef"=w24, "Control Cluster"=w21) -> ()  [unwired: 9 in]
  n439 = node-c288(i64 50 ("Period")) -> (w26:T8)  [unwired: 3 in]
  n440 = timed-loop {
    timing: w26 -> [_]
    timing-out: [_] -> w25
    tunnel: w34 -> [w841]
    tunnel: w21 -> [w837]
    tunnel: w21 -> [w834]
    stop <- _ stop-if-true
    n441 = node-c288() -> (→"Finished Late? [i-1]":bool)  [unwired: 1 in, 1 out]
    n442 = disable-structure shown="Disabled" {
      disable-tunnel: w834 -> [w843 _]
      disable-tunnel: T34 {"Yaw, Driving Straight"={"proportional gain (Kc)"=1.0, "integral time (Ti, min)"=0.01, "derivative time (Td, min)"=0.0}, "Yaw, Holding Still"={"proportional gain (Kc)"=1.0, "integral time (Ti, min)"=0.01, "derivative time (Td, min)"=0.0}, "Distance, Driving Straight"={"proportional gain (Kc)"=1.0, "integral time (Ti, min)"=0.01, "derivative time (Td, min)"=0.0}, "Distance, Holding Still"={"proportional gain (Kc)"=1.0, "integral time (Ti, min)"=0.01, "derivative time (Td, min)"=0.0}} ("PID Gains") -> [w842 _]
      frame Disabled {
        n443 = call <userlib>:"Drive_Loop_PID_Update.vi"("PID Gains"=w842, "Control Cluster"=w843) -> ()  [unwired: 10 in]
      }
      frame Enabled {
      }
    }
    n444 = call <vilib>:"WPI_JoystickGetValues.vi"("JoystickDevRef"=w841) -> ("Axes"=w840:dbl[])  [unwired: 6 in, 4 out]
    n445 = Index Array(array=w840) -> (element #2=w839:dbl, element #3=w838:dbl)  [unwired: 5 in, 3 out]
    n446 = call <userlib>:"Drive_Loop_Cheesey_Drive.vi"("Wheel"=w838, "Throttle"=w839, "Drive Loop Cluster"=w837) -> ()  [unwired: 9 in]
    n447 = node-c288("Period") -> ()  [unwired: 1 out]
  }
  n448 = node-c288(w25) -> ()  [unwired: 1 out]
